vi "LittleEndianToFloat.vi"(11 "Little endian float string":string) -> (3 "Float value":sgl)   [LabVIEW 2020]
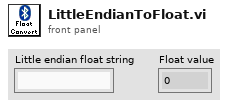
[diagram p1: front panel]
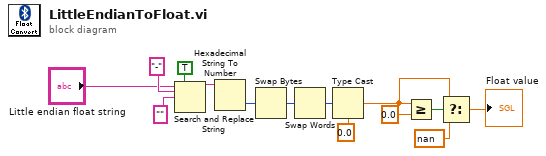
[diagram p0: block diagram]
diagram:
  n1 = Search and Replace String(replace all?=TRUE ("replace all? (F)"), input string="Little endian float string", search string="-", replace string="" ("replace string (\"\")")) -> (result string=w11:string)  [unwired: 4 in, 3 out]
  n2 = Hexadecimal String To Number(string=w11) -> (number=w10:u32)  [unwired: 2 in, 1 out]
  n3 = Swap Bytes(anything=w10) -> (byte swapped=w9:u32)
  n4 = Swap Words(1:w9) -> (0:w8:u32)
  n5 = Type Cast(type=sgl 0.0, x=w8) -> (*(type *) &x=w3:sgl)
  n6 = Greater Or Equal?(x=w3, y=sgl 0.0) -> (x >= y?=w5:bool)
  n7 = Select(t=w3, s=w5, f=sgl nan) -> (s? t:f=→"Float value":sgl)
